vi "flat_top_hann_window.vi"(3 "output control":T1, 4 "data":variant, 5 "X":dbl[](array[numeric]), 6 "a":dbl[](array[numeric])) -> (0 "error out":errorcluster, 1 "f'(X,a)":dbl[][](array[numeric]), 2 "f(X,a)":dbl[](array[numeric]))   [LabVIEW 2019]
doc: "This template is the starting point for creating a model function to be passed to the Nonlinear Curve Fit.vi."
uses:
  <vilib>/gmath/NumericalOptimization/LM_output select.ctl
  <vilib>/gmath/NI_Gmath.lvlib
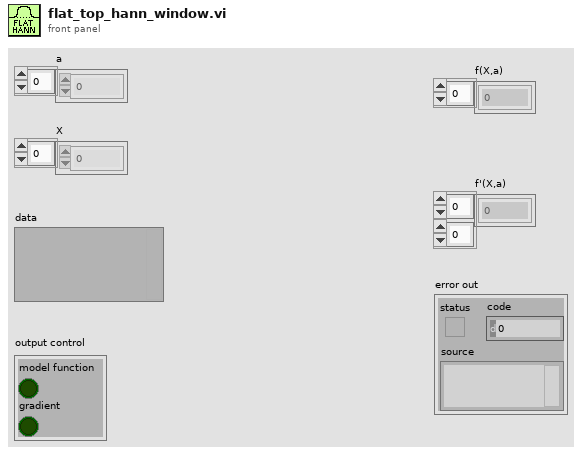
[diagram p1: front panel]
types:
  T1 = typedef "NI_Gmath.lvlib/LM_output select.ctl" = cluster{"model function":bool, "gradient":bool}
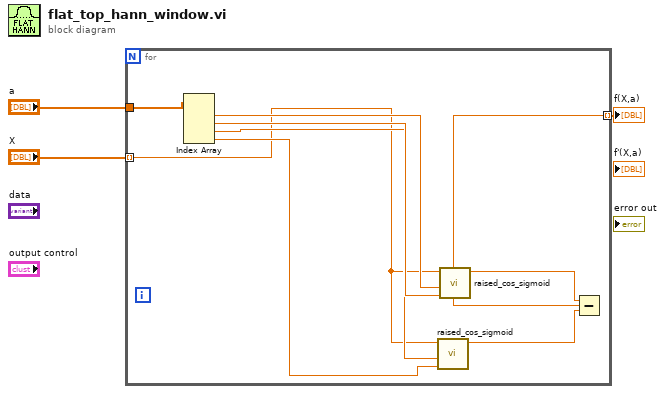
[diagram p0: block diagram]
diagram:
  n1 = for {
    tunnel: "a" -> [w12]
    tunnel: "X" -> [w6] mode=indexing
    tunnel: [w7] -> w1 mode=indexing
    n2 = Index Array(array=w12) -> (element #1=w11:dbl, element #2=w10:dbl, element #3=w9:dbl, element #4=w8:dbl)  [unwired: 4 in]
    n3 = call "raised_cos_sigmoid.vi"("B"=w8, "A"=w9, "x"=w6) -> ("raised_cos_sigmoid(x, A, B)"=w5:dbl)  [unwired: 8 in]
    n4 = call "raised_cos_sigmoid.vi"("B"=w10, "A"=w11, "x"=w6) -> ("raised_cos_sigmoid(x, A, B)"=w4:dbl)  [unwired: 8 in]
    n5 = Subtract(x=w4, y=w5) -> (x-y=w7:dbl)
  }
  "f(X,a)" <- w1
